vi "Two Button Dialog with Timeout.vi"(0 "message":string, 1 "T Timeout(-1 s)":i32=-1, 2 "T button name (\"OK\")":string="OK", 3 "F button name (\"Cancel\")":string="Cancel", 4 "F Timeout(-1 s)":i32=-1, 5 "Parent Wnd(Caller By Default)":refnum<vi>) -> (7 "T button?":bool)   [LabVIEW 2017]
doc: "Shows a two-button dialog carrying the message and the button names given, each button with its own timeout. Returns TRUE when the true button was pressed, and FALSE for the false button or a timeout."
uses:
  a539abf7-d72e-4e1a-867b-c48a8ed28406.vi
  a000c3c0-17f0-4be0-b5ae-7b04c78b6241.vi
  7f025491-3c73-41eb-90d8-dc68797bdda8.vi
panel:
  out "font":T1
  in  "Cancel":bool
  in  "OK":bool
  out "String":string
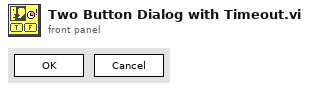
[diagram p1: front panel]
types:
  T1 = cluster{"Font Name:":string, "Size":i16, "Strikeout?":bool, "Italic?":bool, "Underline?":bool, "Outline?":bool, "Shadow?":bool, "Bold?":bool}
  T2 = typedef "LVFontTypeDef.ctl" = cluster{"Font Name":string, "Size":u16, "Bold":bool, "Italic":bool, "Underline":bool, "Strikeout":bool, "Color":u32}
  T3 = cluster{"left":i16, "top":i16, "right":i16, "bottom":i16}
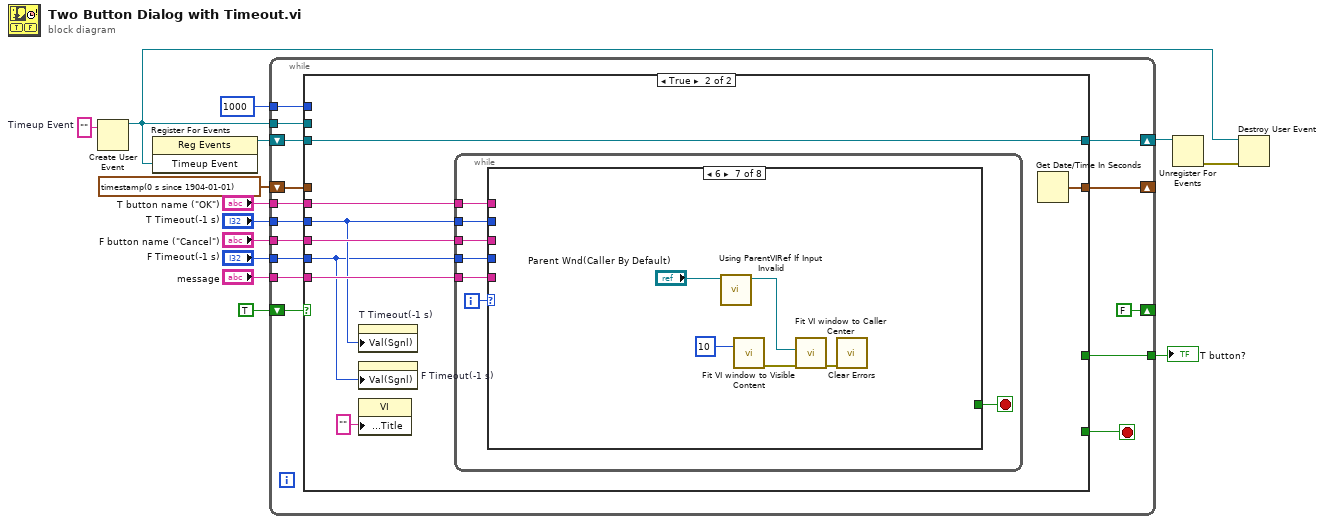
[diagram p0: block diagram]
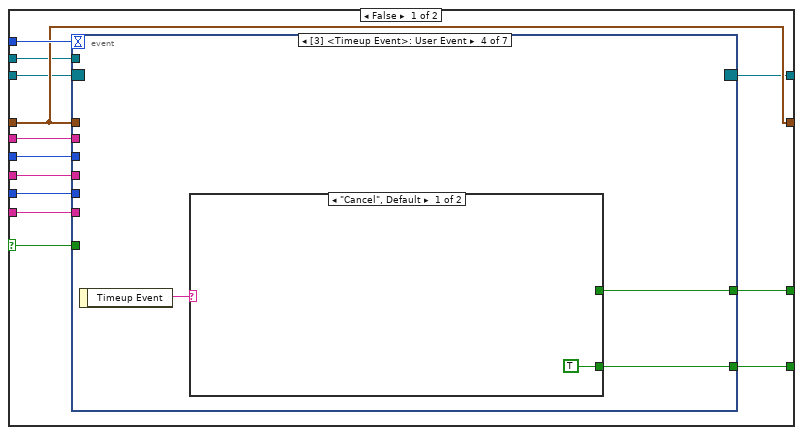
[diagram p2: hidden frame]
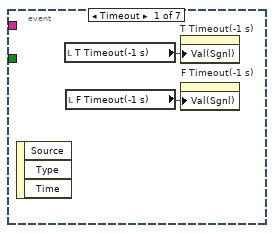
[diagram p3: hidden frame]
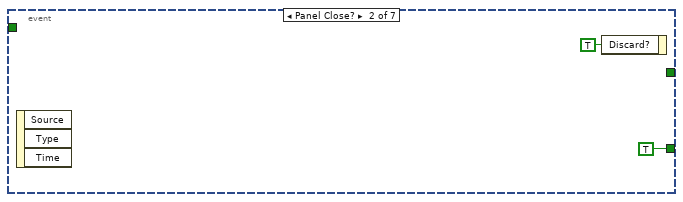
[diagram p4: hidden frame]
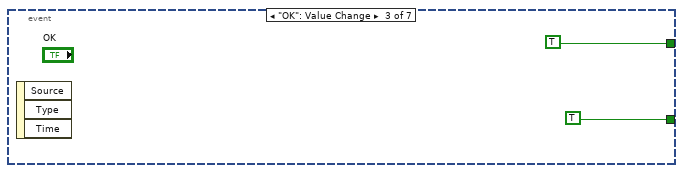
[diagram p5: hidden frame]
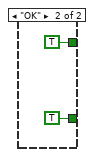
[diagram p6: hidden frame]
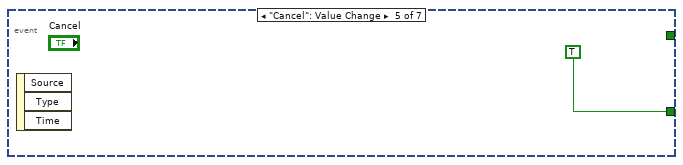
[diagram p7: hidden frame]
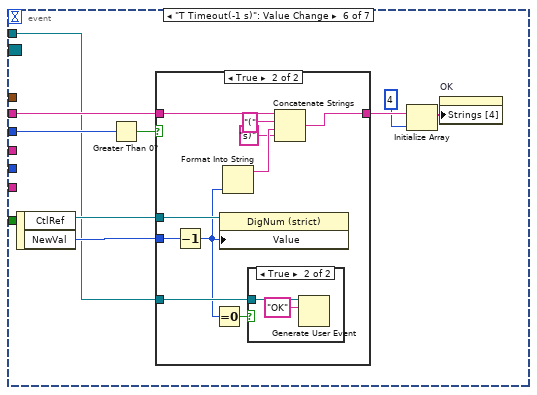
[diagram p8: hidden frame]
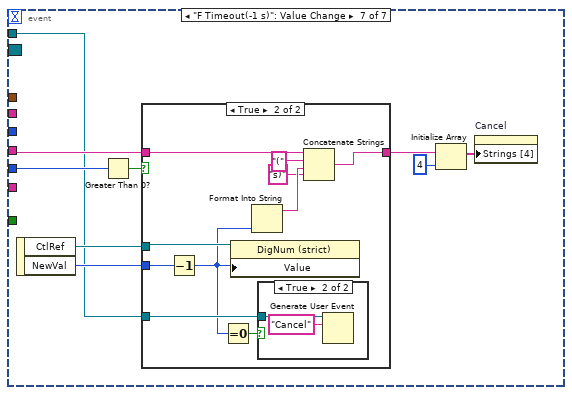
[diagram p11: hidden frame]
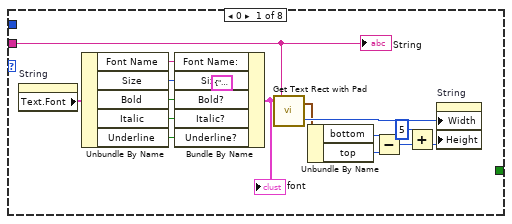
[diagram p14: hidden frame]
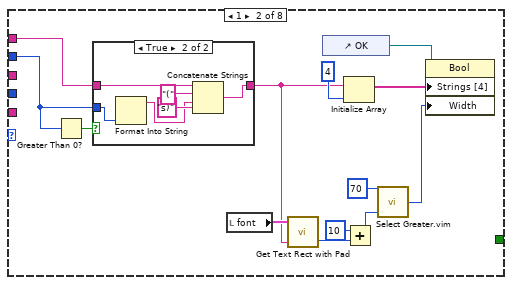
[diagram p15: hidden frame]
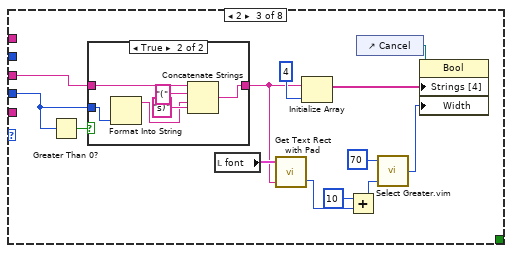
[diagram p17: hidden frame]
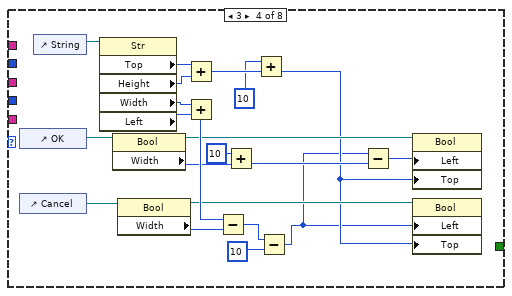
[diagram p19: hidden frame]
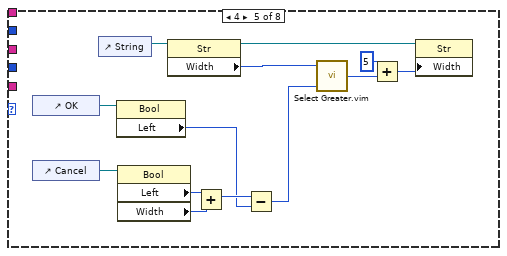
[diagram p20: hidden frame]
diagram:
  w5 = ""  # Timeup Event
  n1 = Create User Event(user event datatype=w5) -> (user event=w1:refnum<user-event>)  [unwired: 1 in, 1 out]
  n2 = register-events(w1) -> (reference out=w4:refnum<event-registration>)  [unwired: 2 in, 1 out]
  n3 = while {
    tunnel: [w28] -> w14
    tunnel: "T button name (\"OK\")" -> [w24]
    tunnel: "F button name (\"Cancel\")" -> [w22]
    tunnel: "message" -> [w25]
    shift-right: [FALSE] -> _
    shift-left: TRUE -> [w27]
    tunnel: "F Timeout(-1 s)" -> [w21]
    tunnel: "T Timeout(-1 s)" -> [w23]
    shift-right: [w20] -> _
    shift-left: timestamp(0 s since 1904-01-01) ("seconds since 1Jan1904") -> [w19]
    tunnel: 1000 -> [w18]
    shift-right: [w16] -> w3
    shift-left: w4 -> [w17]
    tunnel: w1 -> [w15]
    stop <- w29 stop-if-true
    n4 = case shown="True" w27 {
      selector: w27 -> [w39 _]
      tunnel: [w42 _] -> w29
      tunnel: [w41 _] -> w28
      tunnel: w18 -> [w40 _]
      tunnel: w25 -> [w34 w105]
      tunnel: w24 -> [w38 w103]
      tunnel: w23 -> [w37 w102]
      tunnel: w22 -> [w36 w104]
      tunnel: w21 -> [w35 w101]
      tunnel: [w33 w107] -> w20
      tunnel: w19 -> [w33 _]
      tunnel: w17 -> [w32 w106]
      tunnel: [w31 w106] -> w16
      tunnel: w15 -> [w30 _]
      frame False {
        n5 = event shown="[3] <Timeup Event>: User Event" {
          selector: w32 -> [_ _ _ _ _ _ _]
          dyn-events: [_ _ _ _ _ _ _] -> w31
          timeout: w40 -> [_ _ _ _ _ _ _]
          tunnel: [_ TRUE ("Discard?") TRUE ("Discard?") w50 TRUE ("Discard?") _ _] -> w42
          tunnel: [_ _ TRUE w49 _ _ _] -> w41
          tunnel: w39 -> [_ _ _ _ _ _ _]
          tunnel: w38 -> [_ _ _ _ _ w64 _]
          tunnel: w37 -> [_ _ _ _ _ w62 _]
          tunnel: w36 -> [_ _ _ _ _ _ w82]
          tunnel: w35 -> [_ _ _ _ _ _ w81]
          tunnel: w34 -> [_ _ _ _ _ _ _]
          tunnel: w33 -> [_ _ _ _ _ _ _]
          tunnel: w30 -> [_ _ _ _ _ w56 w78]
          event Timeout {
            n6 = event-data() -> ()  [unwired: 1 in, 3 out]
            n7 = local read "T Timeout(-1 s)"() -> (w43:i32)
            n8 = local read "F Timeout(-1 s)"() -> (w44:i32)
            n9 = property on="T Timeout(-1 s)" class="DigNum (strict)"("Val(Sgnl)"=w43) -> ()  [unwired: 2 in, 2 out]
            n10 = property on="F Timeout(-1 s)" class="DigNum (strict)"("Val(Sgnl)"=w44) -> ()  [unwired: 2 in, 2 out]
          }
          event Panel Close? {
            n11 = event-data() -> ()  [unwired: 1 in, 3 out]
            n12 = event-data("Discard?"=TRUE) -> ()  [unwired: 1 in, 1 out]
          }
          event "OK": Value Change {
            n13 = event-data() -> ()  [unwired: 1 in, 3 out]
          }
          event User Event {
            n14 = event-data() -> ("Timeup Event"=w51:string)  [unwired: 1 in]
            n15 = case shown="\"Cancel\", Default" w51 {
              tunnel: [TRUE ("Discard?") TRUE ("Discard?")] -> w50
              tunnel: [_ TRUE ("Discard?")] -> w49
              frame "Cancel", Default {
              }
              frame "OK" {
              }
            }
          }
          event "Cancel": Value Change {
            n16 = event-data() -> ()  [unwired: 1 in, 3 out]
          }
          event "T Timeout(-1 s)": Value Change {
            n17 = event-data() -> ("CtlRef"=w58:refnum<vi>, "NewVal"=w57:i32)  [unwired: 1 in]
            n18 = Greater Than 0?(x=w62) -> (x > 0?=w63:bool)
            n19 = case shown="True" w63 {
              tunnel: w64 -> [w65 w75]
              tunnel: [w65 w71] -> w61
              tunnel: w57 -> [_ w70]
              tunnel: w58 -> [_ w69]
              tunnel: w56 -> [_ w67]
              frame False {
              }
              frame True {
                n20 = Decrement(x=w70) -> (x-1=w66:i32)
                n21 = Equal To 0?(x=w66) -> (x = 0?=w68:bool)
                n22 = property class="DigNum (strict)"(reference=w69, "Value"=w66) -> ()  [unwired: 1 in, 2 out]
                n23 = Format Into String(w66) -> (resulting string=w74:string)  [unwired: 3 in, 1 out]
                n24 = case shown="True" w68 {
                  tunnel: w67 -> [_ w77]
                  frame False {
                  }
                  frame True {
                    n25 = Generate User Event(user event=w77, event data cluster="OK" ("event data")) -> ()  [unwired: 2 in, 2 out]
                  }
                }
                n26 = Concatenate Strings(w75, "(" ("string"), w74, "s)" ("string")) -> (w71:string)
              }
            }
            n27 = Initialize Array(w61, 4 ("dimension size")) -> (w60:string[])
            n28 = property on="OK" class="Bool"("Strings [4]"=w60) -> ()  [unwired: 2 in, 2 out]
          }
          event "F Timeout(-1 s)": Value Change {
            n29 = event-data() -> ("CtlRef"=w80:refnum<vi>, "NewVal"=w79:i32)  [unwired: 1 in]
            n30 = Greater Than 0?(x=w81) -> (x > 0?=w86:bool)
            n31 = case shown="True" w86 {
              tunnel: w82 -> [w87 w97]
              tunnel: [w87 w93] -> w85
              tunnel: w79 -> [_ w92]
              tunnel: w80 -> [_ w91]
              tunnel: w78 -> [_ w89]
              frame False {
              }
              frame True {
                n32 = Decrement(x=w92) -> (x-1=w88:i32)
                n33 = Equal To 0?(x=w88) -> (x = 0?=w90:bool)
                n34 = property class="DigNum (strict)"(reference=w91, "Value"=w88) -> ()  [unwired: 1 in, 2 out]
                n35 = Format Into String(w88) -> (resulting string=w96:string)  [unwired: 3 in, 1 out]
                n36 = case shown="True" w90 {
                  tunnel: w89 -> [_ w99]
                  frame False {
                  }
                  frame True {
                    n37 = Generate User Event(user event=w99, event data cluster="Cancel" ("event data")) -> ()  [unwired: 2 in, 2 out]
                  }
                }
                n38 = Concatenate Strings(w97, "(" ("string"), w96, "s)" ("string")) -> (w93:string)
              }
            }
            n39 = Initialize Array(w85, 4 ("dimension size")) -> (w84:string[])
            n40 = property on="Cancel" class="Bool"("Strings [4]"=w84) -> ()  [unwired: 2 in, 2 out]
          }
        }
      }
      frame True {
        n41 = property on="T Timeout(-1 s)" class="DigNum (strict)"("Val(Sgnl)"=w102) -> ()  [unwired: 2 in, 2 out]
        n42 = property on="F Timeout(-1 s)" class="DigNum (strict)"("Val(Sgnl)"=w101) -> ()  [unwired: 2 in, 2 out]
        n43 = property class="VI"("Front Panel.Title"="" ("Front Panel Window:Title")) -> ()  [unwired: 2 in, 2 out]
        n44 = while {
          tunnel: w105 -> [w114]
          tunnel: w104 -> [w111]
          tunnel: w103 -> [w110]
          tunnel: w102 -> [w109]
          tunnel: w101 -> [w108]
          i -> [w113]
          stop <- w112 stop-if-true
          n45 = case shown="6" w113 {
            tunnel: w114 -> [w129 _ _ _ _ _ _ _]
            tunnel: [_ _ _ _ _ _ _ TRUE] -> w112
            tunnel: w111 -> [_ _ w159 _ _ _ _ _]
            tunnel: w110 -> [_ w140 _ _ _ _ _ _]
            tunnel: w109 -> [_ w139 _ _ _ _ _ _]
            tunnel: w108 -> [_ _ w158 _ _ _ _ _]
            frame 0 {
              n46 = property on="String" class="Str"() -> ("Text.Font"=w130:T2)  [unwired: 2 in, 2 out]
              n47 = Unbundle By Name(w130) -> ("Font Name"=w126:string, "Size"=w125:u16, "Bold"=w124:bool, "Italic"=w122:bool, "Underline"=w123:bool)
              n48 = Bundle By Name(cluster=T1 {"Font Name:"="", "Size"=0, "Strikeout?"=FALSE, "Italic?"=FALSE, "Underline?"=FALSE, "Outline?"=FALSE, "Shadow?"=FALSE, "Bold?"=FALSE} ("Font"), "Font Name:"=w126, "Size"=w125, "Bold?"=w124, "Italic?"=w122, "Underline?"=w123) -> (w127:T1)
              "font" <- w127
              n49 = call "Get Text Rect with Pad.vi"("Text"=w129, "Font"=w127) -> ("Width"=w121:i16, "Rect"=w120:T3)  [unwired: 1 in]
              n50 = Unbundle By Name(w120) -> ("bottom"=w117:i16, "top"=w119:i16)
              n51 = Subtract(x=w117, y=w119) -> (x-y=w118:i16)
              n52 = Add(x=i16 5, y=w118) -> (x+y=w116:i16)
              n53 = property on="String" class="Str"("Width"=w121, "Height"=w116) -> ()  [unwired: 2 in, 2 out]
              "String" <- w129
            }
            frame 1 {
              n54 = Greater Than 0?(x=w139) -> (x > 0?=w143:bool)
              n55 = case shown="True" w143 {
                tunnel: w140 -> [w144 w150]
                tunnel: [w144 w147] -> w136
                tunnel: w139 -> [_ w145]
                frame False {
                }
                frame True {
                  n56 = Format Into String(w145) -> (resulting string=w146:string)  [unwired: 3 in, 1 out]
                  n57 = Concatenate Strings(w150, "(" ("string"), w146, "s)" ("string")) -> (w147:string)
                }
              }
              n58 = local read "font"() -> (w137:T1)
              n59 = call "Get Text Rect with Pad.vi"("Text"=w136, "Font"=w137) -> ("Width"=w135:i16)  [unwired: 1 in, 1 out]
              n60 = control-ref of="OK"() -> (w138:refnum<vi>)
              n61 = Initialize Array(w136, 4 ("dimension size")) -> (w142:string[])
              n62 = Add(x=i16 10, y=w135) -> (x+y=w132:i16)
              n63 = call "Select Greater.vim"("A"=70, "B"=w132) -> ("lesser"=w131:i32)  [unwired: 3 in]
              n64 = property on="Property Node" class="Bool"(reference=w138, "Strings [4]"=w142, "Width"=w131) -> ()  [unwired: 1 in, 2 out]
            }
            frame 2 {
              n65 = Greater Than 0?(x=w158) -> (x > 0?=w163:bool)
              n66 = case shown="True" w163 {
                tunnel: w159 -> [w164 w170]
                tunnel: [w164 w167] -> w156
                tunnel: w158 -> [_ w165]
                frame False {
                }
                frame True {
                  n67 = Format Into String(w165) -> (resulting string=w166:string)  [unwired: 3 in, 1 out]
                  n68 = Concatenate Strings(w170, "(" ("string"), w166, "s)" ("string")) -> (w167:string)
                }
              }
              n69 = local read "font"() -> (w157:T1)
              n70 = call "Get Text Rect with Pad.vi"("Text"=w156, "Font"=w157) -> ("Width"=w154:i16)  [unwired: 1 in, 1 out]
              n71 = Initialize Array(w156, 4 ("dimension size")) -> (w162:string[])
              n72 = Add(x=i16 10, y=w154) -> (x+y=w152:i16)
              n73 = control-ref of="Cancel"() -> (w160:refnum<vi>)
              n74 = call "Select Greater.vim"("A"=70, "B"=w152) -> ("lesser"=w151:i32)  [unwired: 3 in]
              n75 = property on="Property Node" class="Bool"(reference=w160, "Strings [4]"=w162, "Width"=w151) -> ()  [unwired: 1 in, 2 out]
            }
            frame 3 {
              n76 = control-ref of="OK"() -> (w182:refnum<vi>)
              n77 = control-ref of="Cancel"() -> (w184:refnum<vi>)
              n78 = control-ref of="String"() -> (w191:refnum<vi>)
              n79 = property class="Str"(reference=w191) -> ("Top"=w190:i32, "Height"=w189:u32, "Width"=w187:u32, "Left"=w186:i32)  [unwired: 1 in, 2 out]
              n80 = property class="Bool"(reference=w182) -> (reference out=w177:refnum<vi>, "Width"=w181:u32)  [unwired: 1 in, 1 out]
              n81 = property class="Bool"(reference=w184) -> (reference out=w176:refnum<vi>, "Width"=w183:u32)  [unwired: 1 in, 1 out]
              n82 = Add(x=w190, y=w189) -> (x+y=w188:u32)
              n83 = Add(x=w187, y=w186) -> (x+y=w185:u32)
              n84 = Subtract(x=w185, y=w183) -> (x-y=w172:u32)
              n85 = Add(x=u32 10, y=w181) -> (x+y=w180:u32)
              n86 = Add(x=u32 10, y=w188) -> (x+y=w175:u32)
              n87 = Subtract(x=w172, y=u32 10 ("x")) -> (x-y=w171:u32)
              n88 = Subtract(x=w171, y=w180) -> (x-y=w178:u32)
              n89 = property class="Bool"(reference=w177, "Left"=w178, "Top"=w175) -> ()  [unwired: 1 in, 2 out]
              n90 = property class="Bool"(reference=w176, "Left"=w171, "Top"=w175) -> ()  [unwired: 1 in, 2 out]
            }
            frame 4 {
              n91 = control-ref of="OK"() -> (w202:refnum<vi>)
              n92 = control-ref of="Cancel"() -> (w203:refnum<vi>)
              n93 = control-ref of="String"() -> (w204:refnum<vi>)
              n94 = property class="Bool"(reference=w202) -> ("Left"=w197:i32)  [unwired: 1 in, 2 out]
              n95 = property class="Bool"(reference=w203) -> ("Left"=w199:i32, "Width"=w200:u32)  [unwired: 1 in, 2 out]
              n96 = property class="Str"(reference=w204) -> (reference out=w201:refnum<vi>, "Width"=w194:u32)  [unwired: 1 in, 1 out]
              n97 = Add(x=w199, y=w200) -> (x+y=w198:u32)
              n98 = Subtract(x=w198, y=w197) -> (x-y=w193:u32)
              n99 = call "Select Greater.vim"("A"=w194, "B"=w193) -> ("lesser"=w192:u32)  [unwired: 3 in]
              n100 = Add(x=i16 5, y=w192) -> (x+y=w195:u32)
              n101 = property class="Str"(reference=w201, "Width"=w195) -> ()  [unwired: 1 in, 2 out]
            }
            frame 5 {
              n102 = control-ref of="OK"() -> (w216:refnum<vi>)
              n103 = control-ref of="Cancel"() -> (w218:refnum<vi>)
              n104 = control-ref of="String"() -> (w225:refnum<vi>)
              n105 = property class="Str"(reference=w225) -> ("Top"=w224:i32, "Height"=w223:u32, "Width"=w221:u32, "Left"=w220:i32)  [unwired: 1 in, 2 out]
              n106 = property class="Bool"(reference=w216) -> (reference out=w211:refnum<vi>, "Width"=w215:u32)  [unwired: 1 in, 1 out]
              n107 = property class="Bool"(reference=w218) -> (reference out=w210:refnum<vi>, "Width"=w217:u32)  [unwired: 1 in, 1 out]
              n108 = Add(x=w224, y=w223) -> (x+y=w222:u32)
              n109 = Add(x=w221, y=w220) -> (x+y=w219:u32)
              n110 = Subtract(x=w219, y=w217) -> (x-y=w206:u32)
              n111 = Add(x=u32 10, y=w215) -> (x+y=w214:u32)
              n112 = Add(x=u32 10, y=w222) -> (x+y=w209:u32)
              n113 = Subtract(x=w206, y=u32 10 ("x")) -> (x-y=w205:u32)
              n114 = Subtract(x=w205, y=w214) -> (x-y=w212:u32)
              n115 = property class="Bool"(reference=w211, "Left"=w212, "Top"=w209) -> ()  [unwired: 1 in, 2 out]
              n116 = property class="Bool"(reference=w210, "Left"=w205, "Top"=w209) -> ()  [unwired: 1 in, 2 out]
            }
            frame 6 {
              n117 = call "Using ParentVIRef If Input Invalid.vi"("VI Ref (calling VI)"="Parent Wnd(Caller By Default)") -> ("VI Ref"=w226:refnum<vi>)  [unwired: 5 in, 1 out]
              n118 = call "Fit VI window to Visible Content.vi"("border spacing (2 px)"=10) -> ("error out"=w230:errorcluster)  [unwired: 5 in, 1 out]
              n119 = call "Fit VI window to Caller Center.vi"("Error In"=w230, "Background VI Ref (Callee's Caller)"=w226) -> ("Error Out"=w229:errorcluster)  [unwired: 4 in, 1 out]
              n120 = call <vilib>:"Clear Errors.vi"("error in (no error)"=w229) -> ()  [unwired: 5 in, 2 out]
            }
            frame Default {
            }
          }
        }
        n121 = Get Date/Time In Seconds() -> (seconds since 1Jan1904=w107:timestamp)
      }
    }
  }
  "T button?" <- w14
  n122 = Unregister For Events(event registration refnum=w3) -> (error out=w2:errorcluster)  [unwired: 1 in]
  n123 = Destroy User Event(user event=w1, error in=w2) -> ()  [unwired: 1 out]
